vi "http upgrade action.vi"(8 "server information":T1, 9 "plugins":T2, 10 "tcp conn":refnum<k5>, 11 "application request in":T4) -> ()   [LabVIEW 2013, in "http responder.lvclass"]
uses:
  http responder.lvclass
  HTTP server/http request.ctl
  HTTP server/http method.ctl
  HTTP headers/http header data.ctl
  http plugins.ctl
  http upgrade callback.ctl
  HTTP server/http server info.ctl
  http upgrade data.ctl
  HTTP server/Basic HTTP server.lvclass
  HTTP headers/http headers.lvlib
panel:
  out "error IO":errorcluster
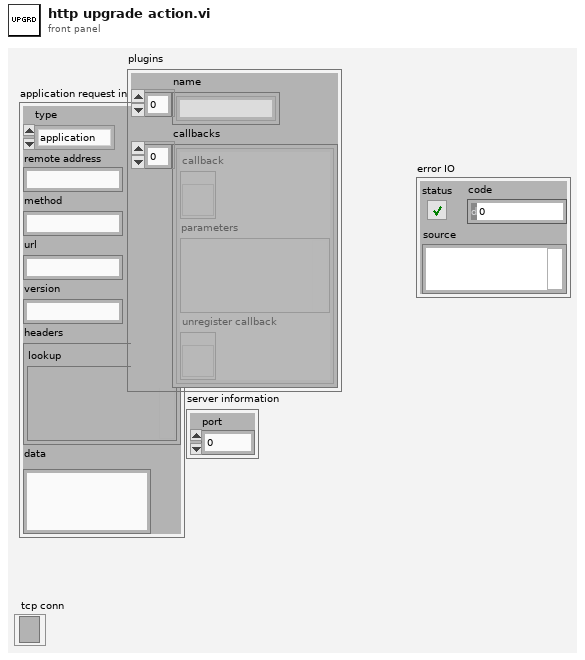
[diagram p1: front panel]
types:
  T1 = typedef "Basic HTTP server.lvclass/http server info.ctl" = cluster{"port":u16}
  T2 = typedef "http responder.lvclass/http plugins.ctl" = cluster{"name":string[], "callbacks":T3[]}
  T3 = typedef "http responder.lvclass/http upgrade callback.ctl" = cluster{"callback":refnum<vi>, "parameters":variant, "unregister callback":refnum<vi>}
  T4 = typedef "Basic HTTP server.lvclass/http request.ctl" = cluster{"type":T5, "remote address":string, "method":string, "url":string, "version":string, "headers":T6, "data":string}
  T5 = typedef "Basic HTTP server.lvclass/http method.ctl" = enum16{"application", "error", "upgrade", "expect"}
  T6 = typedef "http headers.lvlib/http header data.ctl" = cluster{"lookup":variant}
  T7 = typedef "http responder.lvclass/http upgrade data.ctl" = cluster{"TCP connection":refnum<k5>, "application request":T4}
  T8 = typedef "Basic HTTP server.lvclass/http response.ctl" = cluster{"packet type":T9, "reason code":u16, "status string":string, "headers":T6, "cookies":string[], "data":string}
  T9 = typedef "Basic HTTP server.lvclass/http response packet type.ctl" = enum16{"full response", "header only", "data only", "last data", "raw output"}
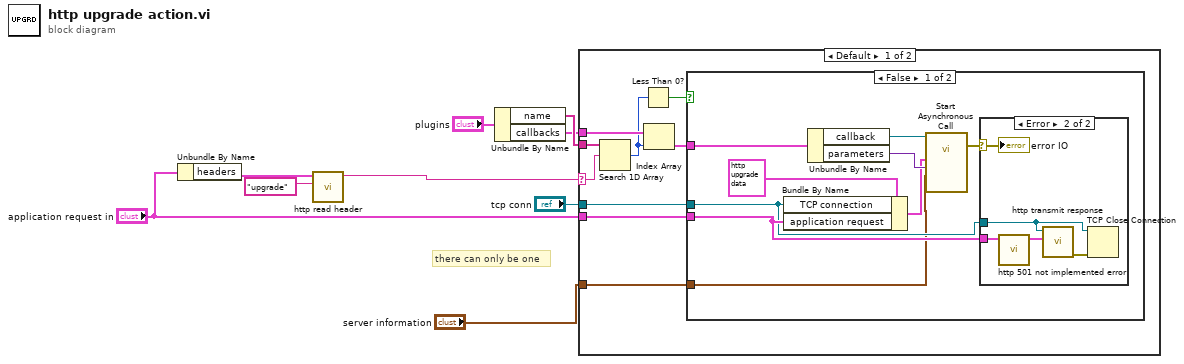
[diagram p0: block diagram]
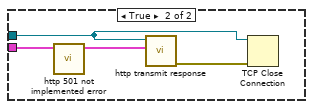
[diagram p3: hidden frame]
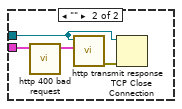
[diagram p4: hidden frame]
diagram:
  # "there can only be one"
  n1 = Unbundle By Name("application request in") -> ("headers"=w3:T6)
  n2 = call "http read header.vi"("header field name"="upgrade" ("name"), "headers"=w3) -> ("value"=w1:string)  [unwired: 8 in, 1 out]
  n3 = Unbundle By Name("plugins") -> ("name"=w6:string[], "callbacks"=w5:T3[])
  n4 = case shown="Default" w1 {
    selector: w1 -> [w14 _]
    tunnel: "tcp conn" -> [w18 w39]
    tunnel: "application request in" -> [w17 w37]
    tunnel: w6 -> [w15 _]
    tunnel: w5 -> [w16 _]
    tunnel: "server information" -> [w10 _]
    frame Default {
      n5 = Search 1D Array(1D array=w15, element=w14) -> (index of element=w12:i32)  [unwired: 1 in]
      n6 = Less Than 0?(x=w12) -> (x < 0?=w11:bool)
      n7 = Index Array(array=w16, index=w12) -> (element=w13:T3)
      n8 = case shown="False" w11 {
        tunnel: w18 -> [w20 w35]
        tunnel: w17 -> [w21 w33]
        tunnel: w13 -> [w27 _]
        tunnel: w10 -> [w19 _]
        frame False {
          n9 = Bundle By Name(cluster=T7 {"TCP connection"=refnum, "application request"={"type"=enum."application", "remote address"="", "method"="", "url"="", "version"="", "headers"={"lookup"=variant}, "data"=""}} ("upgrade data"), "TCP connection"=w20, "application request"=w21) -> (w23:T7)
          n10 = Unbundle By Name(w27) -> ("callback"=w26:refnum<vi>, "parameters"=w25:variant)
          n11 = call-by-ref "Start Asynchronous Call"(reference=w26, "server information"=w19, "parameters"=w25, "upgrade data"=w23) -> (error out=w22:errorcluster)  [unwired: 10 in, 1 out]
          n12 = case shown="Error" w22 {
            selector: w22 -> [_ w28]
            tunnel: w21 -> [_ w30]
            tunnel: w20 -> [_ w29]
            frame No Error {
            }
            frame Error {
              n13 = call "http 501 not implemented error.vi"("application request in"=w30) -> ("application request out"=w31:T8)  [unwired: 10 in]
              n14 = call "http transmit response.vi"("application request"=w31, "tcp connection"=w29) -> ("error out"=w32:errorcluster)  [unwired: 9 in]
              n15 = TCP Close Connection(connection ID=w29, error in (no error)=w32) -> ()  [unwired: 1 in, 2 out]
              "error IO" <- w28
            }
          }
        }
        frame True {
          n16 = call "http 501 not implemented error.vi"("application request in"=w33) -> ("application request out"=w34:T8)  [unwired: 10 in]
          n17 = call "http transmit response.vi"("application request"=w34, "tcp connection"=w35) -> ("error out"=w36:errorcluster)  [unwired: 9 in]
          n18 = TCP Close Connection(connection ID=w35, error in (no error)=w36) -> ()  [unwired: 1 in, 2 out]
        }
      }
    }
    frame "" {
      n19 = call "http 400 bad request.vi"("application request in"=w37) -> ("application request out"=w38:T8)  [unwired: 10 in]
      n20 = call "http transmit response.vi"("application request"=w38, "tcp connection"=w39) -> ("error out"=w40:errorcluster)  [unwired: 9 in]
      n21 = TCP Close Connection(connection ID=w39, error in (no error)=w40) -> ()  [unwired: 1 in, 2 out]
    }
  }
